vi "VoltageDebugFinal.vi"(8 "delay (ms)":u32=500) -> ()   [LabVIEW 2013]
panel:
  out "appended array":string[](array[string])
  in  "VISA PS":refnum<visa-resource-name>="COM1"
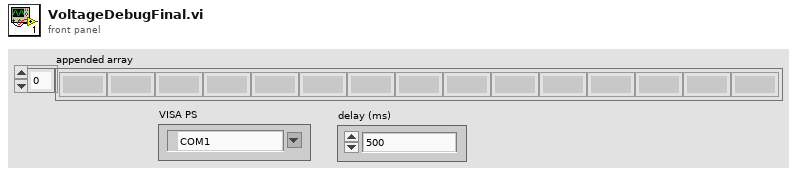
[diagram p1: front panel]
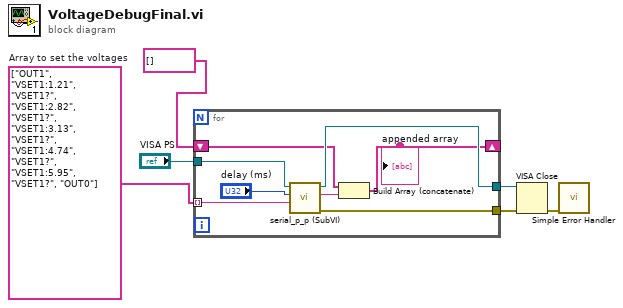
[diagram p0: block diagram]
diagram:
  w4 = string[] ["OUT1", "VSET1:1.21", "VSET1?", "VSET1:2.82", "VSET1?", "VSET1:3.13", "VSET1?", "VSET1:4.74", "VSET1?", "VSET1:5.95", "VSET1?", "OUT0"]  # Array to set the voltages
  n1 = for {
    tunnel: "VISA PS" -> [w13]
    tunnel: w4 -> [w12] mode=indexing
    tunnel: [w9] -> w5
    tunnel: [w10] -> w3
    shift-right: [w7] -> _
    shift-left: string[] [] -> [w8]
    n2 = call "serial_p_p (SubVI).vi"("Command"=w12, "delay before read (ms)"="delay (ms)", "VISA Refnum in"=w13) -> ("error out"=w10:errorcluster, "read buffer"=w11:string, "VISA Refnum out"=w9:refnum<visa-resource-name>)  [unwired: 6 in]
    n3 = Build Array (concatenate)(w8, w11) -> (w7:string[])
    "appended array" <- w7
  }
  n4 = VISA Close(VISA resource name=w5, error in (no error)=w3) -> (error out=w2:errorcluster)
  n5 = call <vilib>:"Simple Error Handler.vi"("error in (no error)"=w2) -> ()  [unwired: 4 in, 5 out]
